vi "Check for Alternative Quadrant Correction.vi"(8 "error in (no error)":errorcluster, 10 "End Point (unreleased)":refnum<class "1D Array f32.lvclass">, 11 "Starting Point (unreleased)":refnum<class "1D Array f32.lvclass">) -> (0 "error out":errorcluster, 3 "Quadrant Correction":refnum<class "1D Array f32.lvclass">)   [LabVIEW 2020, in "G2CPU Line Profile.lvlib"]
uses:
  G2CPU Line Profile.lvlib
  <vilib>/Natan Biesmans/G2CPU GPU and CPU HPC Toolkit/G2CPU Libraries/Arrays/1DArray/f32/1D Array f32.lvclass
  C:/Program Files/National Instruments/LabVIEW 2025/vi.lib/Natan Biesmans/G2CPU GPU and CPU HPC Toolkit/G2CPU Libraries/Arrays/Array/Array Prototype.lvclass
  <vilib>/Natan Biesmans/G2CPU GPU and CPU HPC Toolkit/G2CPU Libraries/Arrays/Array/Array Prototype.lvclass/Array Prototype.ctl
  3b422dd6-199d-4ff1-bfa9-29508a0ffbc1.vi
  cef860aa-4042-46ca-b2f3-709da8d6588c.vi
  41a10666-bec0-4d25-bcb2-2571ea2e3beb.vi
  57ba3f94-8e41-4dbb-8bb7-319169c10130.vi
  <vilib>/Natan Biesmans/G2CPU GPU and CPU HPC Toolkit/G2CPU Libraries/Arrays/Array/G2CPU Get Array Pointer.vi
  3b422dd6-199d-4ff1-bfa9-29508a0ffbc1.vi/2cbae9c5-d993-4013-91e6-67de96abb5a0.vi
  3b422dd6-199d-4ff1-bfa9-29508a0ffbc1.vi/df7b902d-6356-419a-b5d5-2ac54df1e506.vi
  cef860aa-4042-46ca-b2f3-709da8d6588c.vi/e7247370-a01f-465a-ac0e-4dfefcb1bb87.vi
  cef860aa-4042-46ca-b2f3-709da8d6588c.vi/345e91f0-9a5e-4de4-af9c-133346717e4a.vi
  41a10666-bec0-4d25-bcb2-2571ea2e3beb.vi/6197f869-f6d4-49b3-9b2c-cc979b422c2e.vi
  41a10666-bec0-4d25-bcb2-2571ea2e3beb.vi/a7e86dbb-b4c0-485c-89c5-522e60ee265c.vi
  57ba3f94-8e41-4dbb-8bb7-319169c10130.vi/1bf6e03b-eb75-45f6-9764-49dc38a3a024.vi
  57ba3f94-8e41-4dbb-8bb7-319169c10130.vi/2da4419f-02df-47a7-be00-1b7e0871fa33.vi
  3b422dd6-199d-4ff1-bfa9-29508a0ffbc1.vi/df7b902d-6356-419a-b5d5-2ac54df1e506.vi/edd31282-7992-4bba-af75-482693dee5e1.vi
  41a10666-bec0-4d25-bcb2-2571ea2e3beb.vi/6197f869-f6d4-49b3-9b2c-cc979b422c2e.vi/3e802c67-fb96-46a3-ae13-4994a8508b4f.vi
  41a10666-bec0-4d25-bcb2-2571ea2e3beb.vi/6197f869-f6d4-49b3-9b2c-cc979b422c2e.vi/5a50fc67-79e7-4972-80c2-92243cd53dd4.vi
  41a10666-bec0-4d25-bcb2-2571ea2e3beb.vi/6197f869-f6d4-49b3-9b2c-cc979b422c2e.vi/4b7910ad-0c4a-46e4-b1b3-c9721aeaa91e.vi
  41a10666-bec0-4d25-bcb2-2571ea2e3beb.vi/a7e86dbb-b4c0-485c-89c5-522e60ee265c.vi/730f6c57-5c0b-4ee9-b61e-75067b25222b.vi
  41a10666-bec0-4d25-bcb2-2571ea2e3beb.vi/a7e86dbb-b4c0-485c-89c5-522e60ee265c.vi/096b8799-7810-404e-baca-ba9279cec4bd.vi
  41a10666-bec0-4d25-bcb2-2571ea2e3beb.vi/a7e86dbb-b4c0-485c-89c5-522e60ee265c.vi/0f1a5a47-bcc5-4796-ac31-8dfcfbc0d7d1.vi
  41a10666-bec0-4d25-bcb2-2571ea2e3beb.vi/a7e86dbb-b4c0-485c-89c5-522e60ee265c.vi/89f12e17-3330-4b72-ad8f-8dd636660732.vi
  57ba3f94-8e41-4dbb-8bb7-319169c10130.vi/1bf6e03b-eb75-45f6-9764-49dc38a3a024.vi/3e802c67-fb96-46a3-ae13-4994a8508b4f.vi
  57ba3f94-8e41-4dbb-8bb7-319169c10130.vi/1bf6e03b-eb75-45f6-9764-49dc38a3a024.vi/5a50fc67-79e7-4972-80c2-92243cd53dd4.vi
  57ba3f94-8e41-4dbb-8bb7-319169c10130.vi/1bf6e03b-eb75-45f6-9764-49dc38a3a024.vi/4b7910ad-0c4a-46e4-b1b3-c9721aeaa91e.vi
  57ba3f94-8e41-4dbb-8bb7-319169c10130.vi/2da4419f-02df-47a7-be00-1b7e0871fa33.vi/730f6c57-5c0b-4ee9-b61e-75067b25222b.vi
  57ba3f94-8e41-4dbb-8bb7-319169c10130.vi/2da4419f-02df-47a7-be00-1b7e0871fa33.vi/096b8799-7810-404e-baca-ba9279cec4bd.vi
  57ba3f94-8e41-4dbb-8bb7-319169c10130.vi/2da4419f-02df-47a7-be00-1b7e0871fa33.vi/0f1a5a47-bcc5-4796-ac31-8dfcfbc0d7d1.vi
  57ba3f94-8e41-4dbb-8bb7-319169c10130.vi/2da4419f-02df-47a7-be00-1b7e0871fa33.vi/89f12e17-3330-4b72-ad8f-8dd636660732.vi
  <vilib>/Natan Biesmans/G2CPU GPU and CPU HPC Toolkit/ArrayFire Driver/VIs/Run as Multi Device.vi
  41a10666-bec0-4d25-bcb2-2571ea2e3beb.vi/6197f869-f6d4-49b3-9b2c-cc979b422c2e.vi/5a50fc67-79e7-4972-80c2-92243cd53dd4.vi/1b7cf390-2ae0-48f3-9bce-03c57eed6ee8.vi
  57ba3f94-8e41-4dbb-8bb7-319169c10130.vi/1bf6e03b-eb75-45f6-9764-49dc38a3a024.vi/5a50fc67-79e7-4972-80c2-92243cd53dd4.vi/1b7cf390-2ae0-48f3-9bce-03c57eed6ee8.vi
  <vilib>/Natan Biesmans/G2CPU GPU and CPU HPC Toolkit/G2CPU Libraries/Arrays/1DArray/binary/1D Array binary.lvclass
  <vilib>/Natan Biesmans/G2CPU GPU and CPU HPC Toolkit/ArrayFire Driver/VIs/lt.vi
  <vilib>/Natan Biesmans/G2CPU GPU and CPU HPC Toolkit/G2CPU Libraries/Arrays/Array/G2CPU Set Array Pointer.vi
  <vilib>/Natan Biesmans/G2CPU GPU and CPU HPC Toolkit/G2CPU Libraries/Arrays/Array/G2CPU Release Array.vi
  <vilib>/Natan Biesmans/G2CPU GPU and CPU HPC Toolkit/ArrayFire Driver/VIs/cast.vi
  <vilib>/Natan Biesmans/G2CPU GPU and CPU HPC Toolkit/ArrayFire Driver/subvi/Error Converter (ErrCode or Status).vi
  <vilib>/Natan Biesmans/G2CPU GPU and CPU HPC Toolkit/G2CPU Libraries/Arrays/SubVI/is 1D.vi
  <vilib>/Natan Biesmans/G2CPU GPU and CPU HPC Toolkit/ArrayFire Driver/VIs/mul.vi
  <vilib>/Natan Biesmans/G2CPU GPU and CPU HPC Toolkit/ArrayFire Driver/VIs/sub.vi
  <vilib>/Natan Biesmans/G2CPU GPU and CPU HPC Toolkit/G2CPU Libraries/Arrays/1DArray/1D Array Prototype.lvclass
  <vilib>/Natan Biesmans/G2CPU GPU and CPU HPC Toolkit/G2CPU Libraries/Arrays/Array/Array Prototype.lvclass
  <vilib>/Natan Biesmans/G2CPU GPU and CPU HPC Toolkit/G2CPU Libraries/Arrays/DataTypes/f32/f32.lvclass
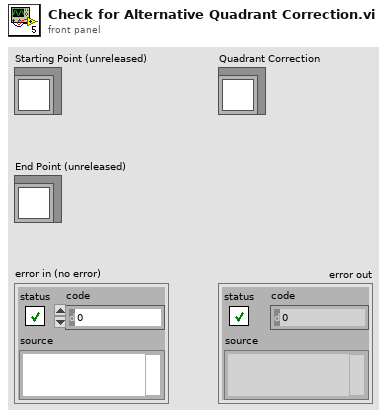
[diagram p1: front panel]
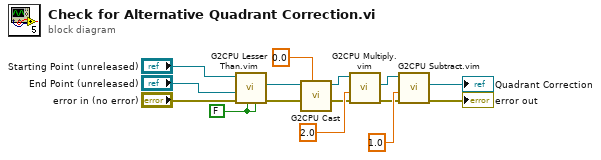
[diagram p0: block diagram]
diagram:
  w11 = FALSE ("Auto Release lhs (Enabled)")
  n1 = call "G2CPU Lesser Than.vim"("Auto Release rhs (Enabled)"=w11, "Auto Release lhs (Enabled)"=w11, "error in (no error)"="error in (no error)", "Array rhs"="End Point (unreleased)", "Array lhs"="Starting Point (unreleased)") -> ("error out"=w5:errorcluster, "Array Result"=w12:refnum<class "1D Array binary.lvclass">)  [unwired: 5 in]
  n2 = call "G2CPU Cast"("Datatype Prototype"=sgl 0.0, "error in (no error)"=w5, "Array In"=w12) -> ("error out"=w4:errorcluster, "Array Out"=w9:refnum<class "1D Array f32.lvclass">)  [unwired: 7 in]
  n3 = call "G2CPU Multiply.vim"("error in (no error)"=w4, "Array rhs"=sgl 2.0 ("Datatype Prototype"), "Array lhs"=w9) -> ("error out"=w3:errorcluster, "Array Result"=w7:refnum<class "1D Array f32.lvclass">)  [unwired: 7 in]
  n4 = call "G2CPU Subtract.vim"("error in (no error)"=w3, "Array rhs"=sgl 1.0 ("Datatype Prototype"), "Array lhs"=w7) -> ("error out"=→"error out":errorcluster, "Array Result"=→"Quadrant Correction":refnum<class "1D Array f32.lvclass">)  [unwired: 7 in]
